vi "Pre-Build Action - Copy (2).vi"(6 "Top Level/Always Included VIs":path[](array[path]), 7 "Main Destination Path":path, 9 "Target Name":string, 10 "Build Specification Name":string, 11 "Project Path":path) -> (0 "error out":errorcluster)   [LabVIEW 2018]
uses:
  <vilib>/AppBuilder/AB_API_Simple/Get Build Specification Version (path).vi
  <vilib>/Utility/config.llb/Write Key (String).vi
  <vilib>/Utility/config.llb/NI_LVConfig.lvlib
  <vilib>/AppBuilder/AB_API_Simple/NI_App_Builder_API.lvlib
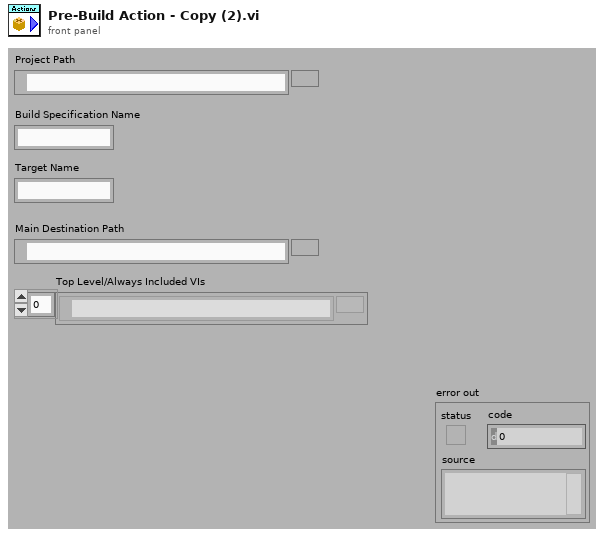
[diagram p1: front panel]
types:
  T1 = typedef "NI_LVConfig.lvlib/Config Data RefNum.ctl" = refnum<k1>
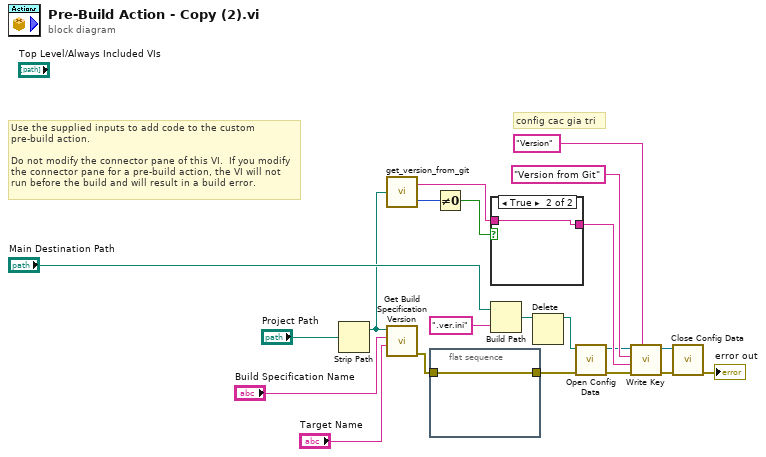
[diagram p0: block diagram]
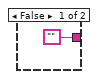
[diagram p2: hidden frame]
diagram:
  # "config cac gia tri"
  # "Use the supplied inputs to add code to the custom pre-build action.\n\nDo not modify the connector pane of this VI.  If you modify the connector pane for a pre-build action, the VI will not run before the build and will result in a build error."
  n1 = Strip Path(path="Project Path") -> (stripped path=w14:path)  [unwired: 1 out]
  n2 = call "get_version_from_git.vi"("path_project"=w14) -> ("Version"=w3:string, "return code"=w5:i32)
  n3 = call-poly <vilib>:"Get Build Specification Version.vi"("Name of target (My Computer)"="Target Name", "Name of build specification"="Build Specification Name", "Path to project"=w14) -> ("error out"=w21:errorcluster)  [unwired: 7 in, 1 out]
  n4 = flat-sequence {
    tunnel: w21 -> [w22]
    tunnel: [w22] -> w2
    frame #0 {
    }
  }
  n5 = Not Equal To 0?(x=w5) -> (x != 0?=w4:bool)
  n6 = case shown="True" w4 {
    tunnel: ["" w24] -> w16
    tunnel: w3 -> [_ w24]
    frame False {
    }
    frame True {
    }
  }
  n7 = Build Path(base path="Main Destination Path", name or relative path=".ver.ini") -> (appended path=w12:path)
  n8 = Delete(path (use dialog)=w12) -> (deleted path=w11:path)  [unwired: 4 in, 2 out]
  n9 = call <vilib>:"Open Config Data.vi"("error in (no error)"=w2, "configuration file path"=w11) -> ("error out"=w6:errorcluster, "refnum"=w10:T1)  [unwired: 1 in, 7 out]
  n10 = call-poly <vilib>:"Write Key.vi"("section"="Version" ("key"), "error in (no error)"=w6, "value"=w16, "key"="Version from Git", "refnum"=w10) -> ("error out"=w7:errorcluster, "refnum out"=w8:T1)  [unwired: 4 in, 1 out]
  n11 = call <vilib>:"Close Config Data.vi"("error in (no error)"=w7, "refnum"=w8) -> ("error out"=→"error out":errorcluster)  [unwired: 8 in, 1 out]
